vi "Apply Size To Object.vi"(7 "properties to ignore":variant, 8 "error in (no error)":errorcluster, 9 "scaling settings":T1={"scaling factor"={"horizontal"=1.0, "vertical"=1.0}, "scale text"=FALSE} {"scaling factor"."vertical" min=0.0; "scaling factor"."horizontal" min=0.0}, 10 "GObj Refnum":refnum<vi>, 11 "NI_SE_Object Layout in":refnum<class "Object Layout.lvclass">) -> (0 "error out":errorcluster, 3 "NI_SE_Object Layout out":refnum<class "Object Layout.lvclass">)   [LabVIEW 2012, in "NI_SE_Front Panel Layout.lvlib" / "Object Layout.lvclass"]
uses:
  Object Layout.lvclass
  Scaling Factor_Options.ctl
  XY Scaling Factor.ctl
  Object Layout.lvclass/Object Layout.ctl
  Properties To Ignore.vi
  NI_SE_Front Panel Layout.lvlib
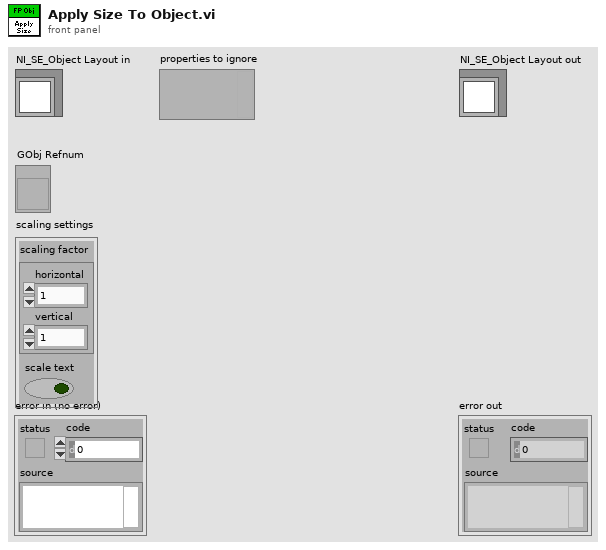
[diagram p1: front panel]
types:
  T1 = typedef "NI_SE_Front Panel Layout.lvlib/Scaling Factor_Options.ctl" = cluster{"scaling factor":T2, "scale text":bool}
  T2 = typedef "NI_SE_Front Panel Layout.lvlib/XY Scaling Factor.ctl" = cluster{"horizontal":dbl, "vertical":dbl}
  T3 = typedef "LVBoundsTypeDef.ctl" = cluster{"Width":u32, "Height":u32}
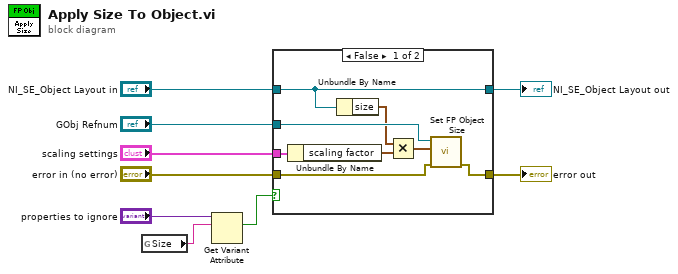
[diagram p0: block diagram]
diagram:
  n1 = global read "Properties To Ignore.vi" "Size"() -> (w1:string)
  n2 = Get Variant Attribute(Variant="properties to ignore", name=w1) -> (found=w2:bool)  [unwired: 2 in, 3 out]
  n3 = case shown="False" w2 {
    tunnel: "error in (no error)" -> [w17 w18]
    tunnel: [w16 w18] -> w8
    tunnel: "NI_SE_Object Layout in" -> [w12 w19]
    tunnel: "scaling settings" -> [w11 _]
    tunnel: "GObj Refnum" -> [w15 _]
    tunnel: [w12 w19] -> w3
    frame False {
      n4 = Unbundle By Name(w11) -> ("scaling factor"=w10:T2)
      n5 = Unbundle By Name(w12) -> ("size"=w14:T3)
      n6 = Multiply(x=w14, y=w10) -> (x*y=w13:T2)
      n7 = call "Set FP Object Size.vi"("error in"=w17, "size"=w13, "object refnum"=w15) -> ("error out"=w16:errorcluster)  [unwired: 7 in, 1 out]
    }
    frame True {
    }
  }
  "error out" <- w8
  "NI_SE_Object Layout out" <- w3
